vi "Frame Update UI From Data.vi"(8 "error in (no error)":errorcluster, 11 "IDE simple in":refnum<class "Main Panel.lvclass">) -> (0 "error out":errorcluster, 3 "IDE simple out":refnum<class "Main Panel.lvclass">)   [LabVIEW 2018, in "Main Panel.lvlib" / "Main Panel.lvclass"]
uses:
  Main Panel.lvclass
  Main Panel.lvclass/Main Panel.ctl
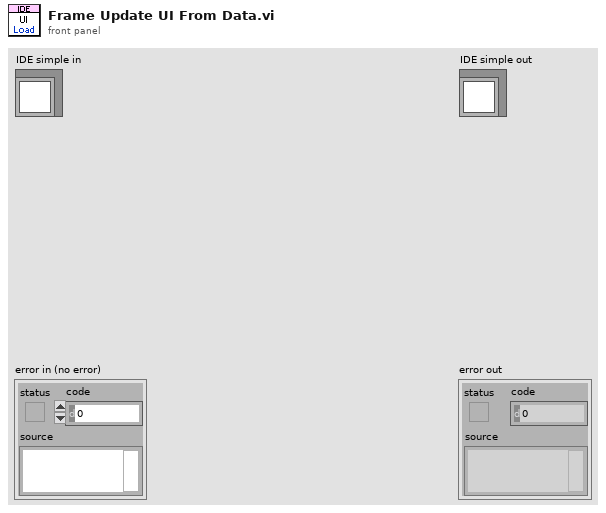
[diagram p1: front panel]
types:
  T1 = typedef "Data Parser.lvclass/frame title.ctl" = cluster{"Number":string, "Name":string}
  T2 = typedef "Data Parser.lvclass/frame basic data.ctl" = cluster{"Basic":cluster{"pic":string, "state":string, "wait":string, "next":string}, "Move":cluster{"dvx":string, "dvy":string, "dvz":string}, "Pic Center":cluster{"centerx":string, "centery":string}, "Skill":cluster{"hit_a":string, "hit_d":string, "hit_j":string, "hit_Fa":string, "hit_Ua":string, "hit_Da":string, "hit_Fj":string, "hit_Uj":string, "hit_Dj":string, "hit_ja":string}, "Mp":string}
  T3 = typedef "Data Parser.lvclass/frame bp data.ctl" = cluster{"x":string, "y":string}
  T4 = typedef "Data Parser.lvclass/frame w data.ctl" = cluster{"kind":string, "x":string, "y":string, "weaponact":string, "dvx":string, "dvy":string, "dvz":string, "attacking":string, "cover":string}
  T5 = typedef "Data Parser.lvclass/frame b data.ctl" = cluster{"kind":string, "x":string, "y":string, "w":string, "h":string}
  T6 = typedef "Data Parser.lvclass/frame i data.ctl" = cluster{"kind":string, "x":string, "y":string, "w":string, "h":string, "dvx":string, "dvy":string, "dvz":string, "fall":string, "arest":string, "vrest":string, "bdefend":string, "injury":string, "zwidth":string, "effect":string, "catchingact":string, "caughtact":string}
  T7 = typedef "Data Parser.lvclass/frame o data.ctl" = cluster{"kind":string, "x":string, "y":string, "action":string, "dvx":string, "dvy":string, "dvz":string, "oid":string, "facing":string}
  T8 = typedef "Data Parser.lvclass/frame c data.ctl" = cluster{"kind":string, "x":string, "y":string, "injury":string, "cover":string, "vaction":string, "aaction":string, "taction":string, "hurtable":string, "decrease":string, "fronthurtact":string, "backhurtact":string, "dircontrol":string, "throwvx":string, "throwvy":string, "throwvz":string, "throwinjury":string}
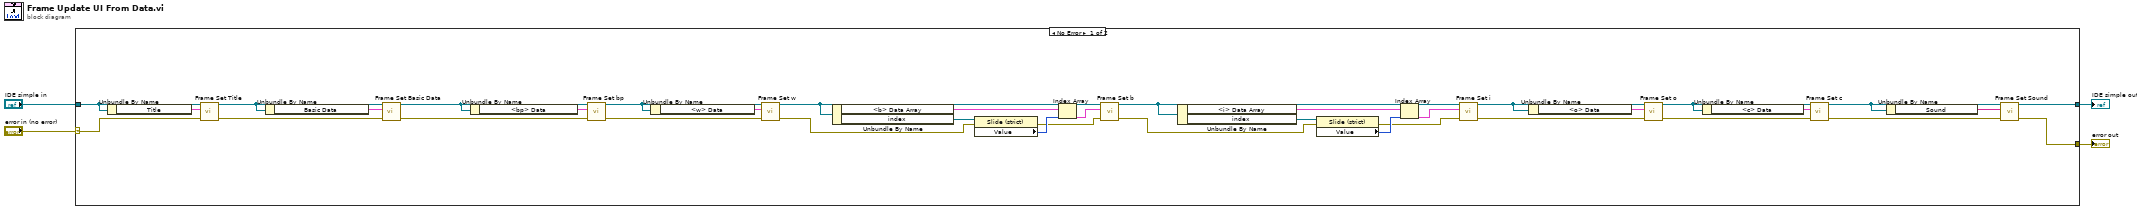
[diagram p0: block diagram]
diagram:
  n1 = case shown="No Error" "error in (no error)" {
    selector: "error in (no error)" -> [w34 w43]
    tunnel: [w5 w43] -> w3
    tunnel: [w6 w42] -> w1
    tunnel: "IDE simple in" -> [w36 w42]
    frame No Error {
      n2 = Unbundle By Name(w36) -> ("Title"=w35:T1)
      n3 = call "Frame Set Title.vi"("error in (no error)"=w34, "Frame Title"=w35, "IDE simple in"=w36) -> ("error out"=w41:errorcluster, "IDE simple out"=w33:refnum<class "Main Panel.lvclass">)  [unwired: 7 in]
      n4 = Unbundle By Name(w33) -> ("Basic Data"=w32:T2)
      n5 = call "Frame Set Basic Data.vi"("error in (no error)"=w41, "Frame Basic Data"=w32, "IDE simple in"=w33) -> ("error out"=w40:errorcluster, "IDE simple out"=w31:refnum<class "Main Panel.lvclass">)  [unwired: 7 in]
      n6 = Unbundle By Name(w31) -> ("<bp> Data"=w30:T3)
      n7 = call "Frame Set bp.vi"("error in (no error)"=w40, "<bp> Data"=w30, "IDE simple in"=w31) -> ("error out"=w39:errorcluster, "IDE simple out"=w29:refnum<class "Main Panel.lvclass">)  [unwired: 7 in]
      n8 = Unbundle By Name(w29) -> ("<w> Data"=w28:T4)
      n9 = call "Frame Set w.vi"("error in (no error)"=w39, "<w> Data"=w28, "IDE simple in"=w29) -> ("error out"=w21:errorcluster, "IDE simple out"=w27:refnum<class "Main Panel.lvclass">)  [unwired: 7 in]
      n10 = Unbundle By Name(w27) -> ("<b> Data Array"=w25:T5[], "index"=w26:refnum<vi>)
      n11 = property class="Slide (strict)"(reference=w26, error in=w21) -> (error out=w22:errorcluster, "Value"=w24:u32)  [unwired: 1 out]
      n12 = Index Array(array=w25, index=w24) -> (element=w23:T5)
      n13 = call "Frame Set b.vi"("error in (no error)"=w22, "<b> Data"=w23, "IDE simple in"=w27) -> ("error out"=w14:errorcluster, "IDE simple out"=w20:refnum<class "Main Panel.lvclass">)  [unwired: 7 in]
      n14 = Unbundle By Name(w20) -> ("<i> Data Array"=w18:T6[], "index"=w19:refnum<vi>)
      n15 = property class="Slide (strict)"(reference=w19, error in=w14) -> (error out=w15:errorcluster, "Value"=w17:u32)  [unwired: 1 out]
      n16 = Index Array(array=w18, index=w17) -> (element=w16:T6)
      n17 = call "Frame Set i.vi"("error in (no error)"=w15, "<i> Data"=w16, "IDE simple in"=w20) -> ("error out"=w38:errorcluster, "IDE simple out"=w13:refnum<class "Main Panel.lvclass">)  [unwired: 7 in]
      n18 = Unbundle By Name(w13) -> ("<o> Data"=w12:T7)
      n19 = call "Frame Set o.vi"("error in (no error)"=w38, "<o> Data"=w12, "IDE simple in"=w13) -> ("error out"=w37:errorcluster, "IDE simple out"=w11:refnum<class "Main Panel.lvclass">)  [unwired: 7 in]
      n20 = Unbundle By Name(w11) -> ("<c> Data"=w10:T8)
      n21 = call "Frame Set c.vi"("error in (no error)"=w37, "<c> Data"=w10, "IDE simple in"=w11) -> ("error out"=w9:errorcluster, "IDE simple out"=w7:refnum<class "Main Panel.lvclass">)  [unwired: 7 in]
      n22 = Unbundle By Name(w7) -> ("Sound"=w8:string)
      n23 = call "Frame Set Sound.vi"("error in (no error)"=w9, "Sound"=w8, "IDE simple in"=w7) -> ("error out"=w5:errorcluster, "IDE simple out"=w6:refnum<class "Main Panel.lvclass">)  [unwired: 7 in]
    }
    frame Error {
    }
  }
  "error out" <- w3
  "IDE simple out" <- w1
